vi "Circus Config Param - Core.vi"(6 "Load":bool, 8 "error in (no error)":errorcluster, 11 "Parameter Name":string) -> (0 "error out":errorcluster, 3 "Output":string)   [LabVIEW 2026, in "TALOS.lvlib"]
doc: "This VI stores in memory all the AEgIS configuration parameters loaded at startup from AEgIS_Config_Param.ini. It only runs when the VI is called from the PPL version of TALOS."
uses:
  TALOS.lvlib
  Ancestor/Ancestor/Ancestor.lvclass/Ancestor.ctl
  FGV/Error Memory/Get Error Description.vi
  Get PC name.vi
  Ancestor/Ancestor/Read ID.vi
  Get Class Name.vi
  <vilib>/Utility/error.llb/Clear Errors.vi
  FGV/Error Memory/Error Memory Core.vi
  <vilib>/AdvancedString/Delimited String to 1D String Array.vi
  <vilib>/AdvancedString/Delimited String to 1D String Array (string).vi
  FGV/Error Memory/Error Crt Lvl checker.vi
  FGV/Error Memory/Error Memory Core.vi/40c8088d-b597-4017-91af-faa98e00292e.vi
  FGV/Error Memory/Error Memory Core.vi/d4a3ab98-063c-4e44-b43d-fbdcfe6c2be2.vi
  Global Memory.vi
  <vilib>/Utility/LVClass/Get LV Class Name.vi
  TALOS Root path.vi
  Read CSV worksheet.vi
  Global Constants.vi
  <vilib>/Utility/error.llb/General Error Handler.vi
  <vilib>/Utility/config.llb/Read Key (String).vi
  Ancestor/Ancestor/Ancestor.lvclass
  <vilib>/Comparison/Equal/Equal Functor/Equal Functor.lvclass
  <vilib>/Utility/config.llb/NI_LVConfig.lvlib
panel:
  out "key names":string[][](array[string])
  out "section names":string[](array[string])
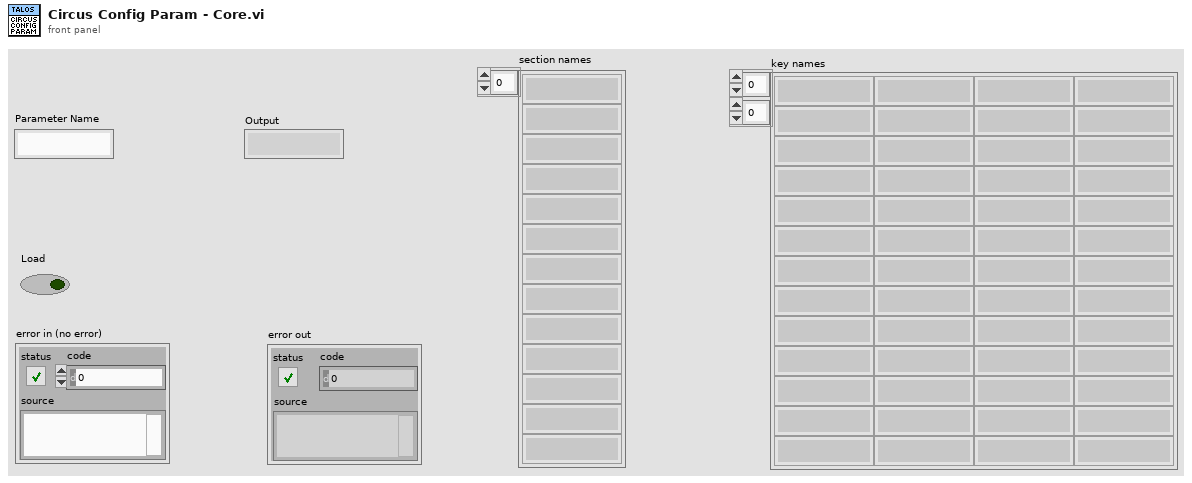
[diagram p1: front panel]
types:
  T1 = typedef "NI_LVConfig.lvlib/Config Data RefNum.ctl" = refnum<k1>
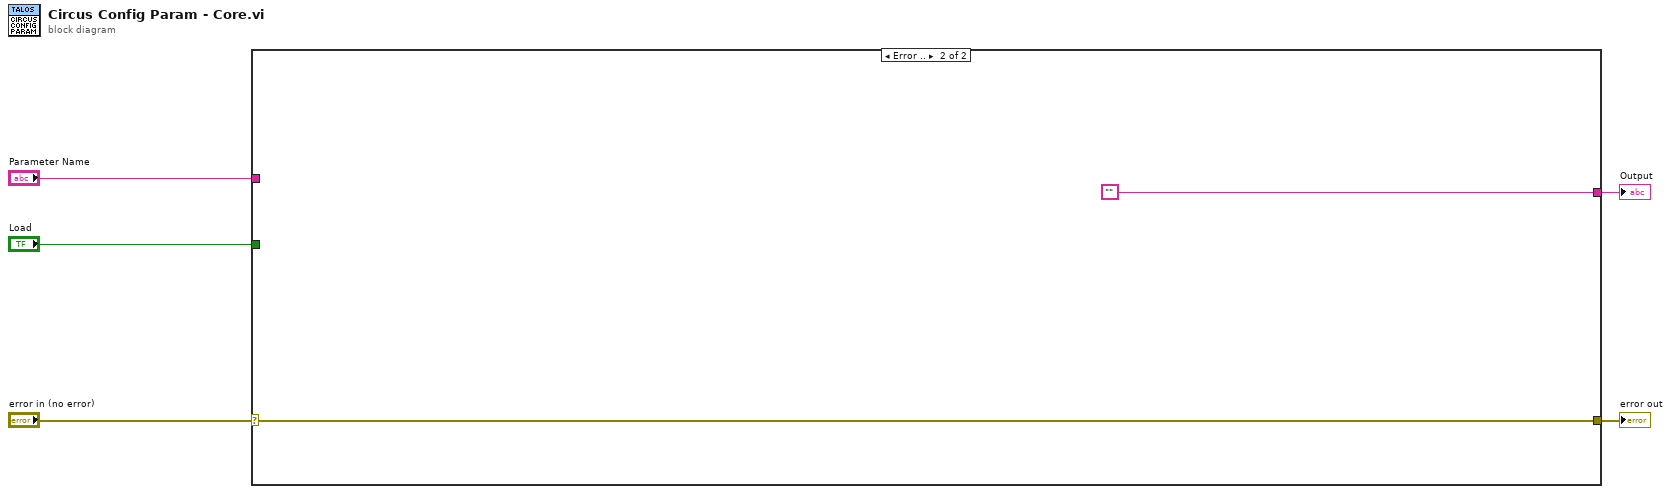
[diagram p0: block diagram]
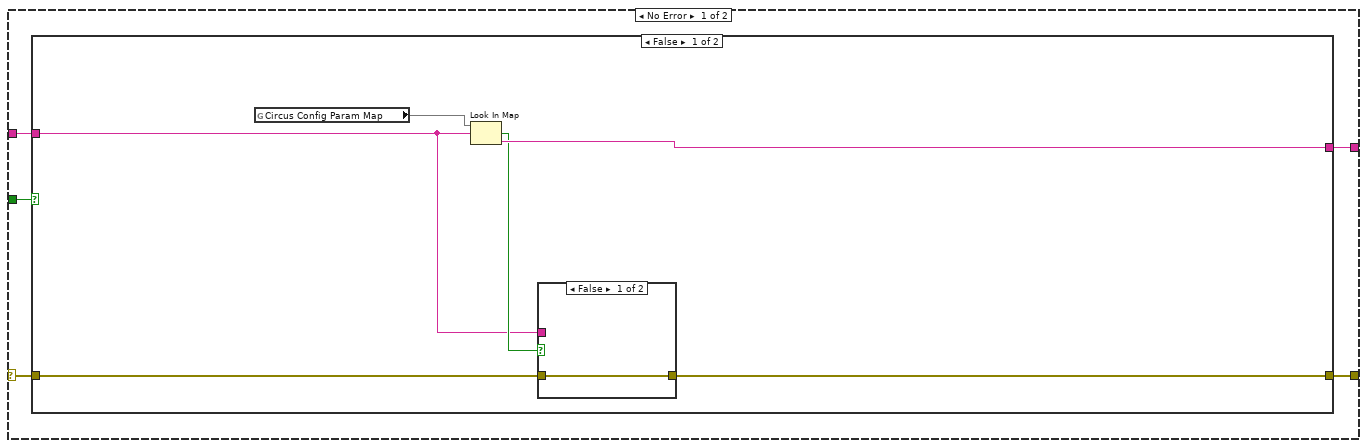
[diagram p2: hidden frame]
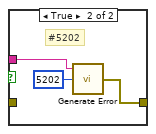
[diagram p3: hidden frame]
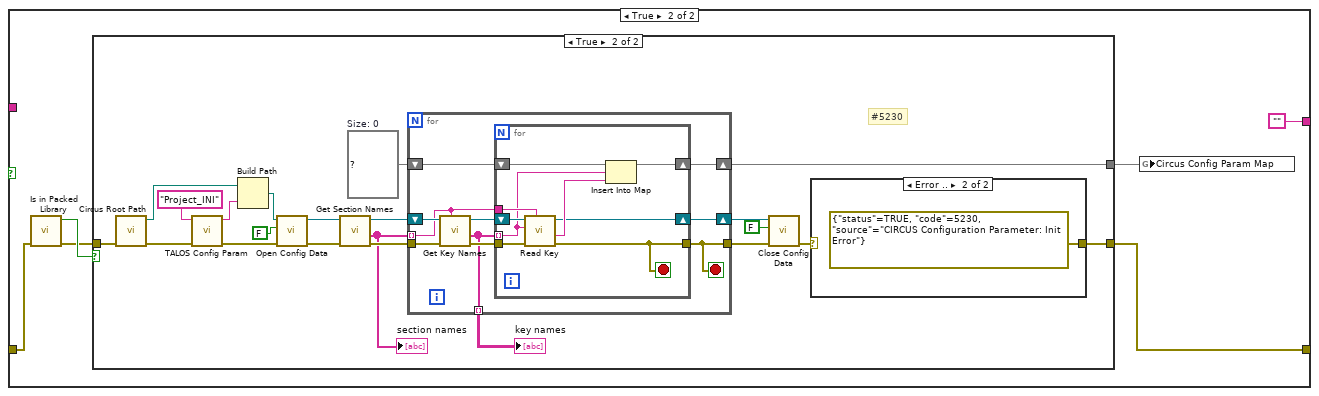
[diagram p4: hidden frame]
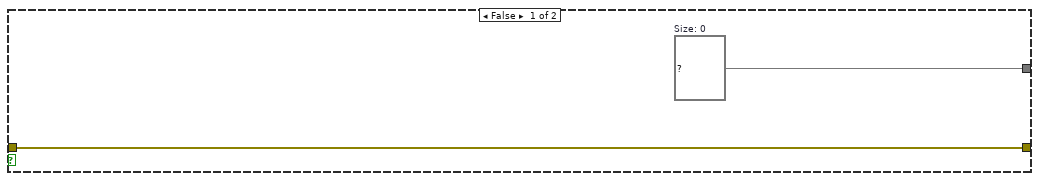
[diagram p5: hidden frame]
diagram:
  n1 = case shown="Error .." "error in (no error)" {
    selector: "error in (no error)" -> [w6 w72]
    tunnel: "Load" -> [w10 _]
    tunnel: [w9 w72] -> w4
    tunnel: [w8 "" ("Empty String Constant")] -> w3
    tunnel: "Parameter Name" -> [w7 _]
    frame No Error {
      n2 = case shown="False" w10 {
        tunnel: w6 -> [w14 w21]
        tunnel: [w13 w26] -> w9
        tunnel: [w16 "" ("Output")] -> w8
        tunnel: w7 -> [w11 _]
        frame False {
          n3 = global read "Global Memory.vi" "Circus Config Param Map"() -> (w12:map{string, string})
          n4 = Look In Map(map=w12, key=w11) -> (key not found?=w15:bool, value=w16:string)  [unwired: 1 in]
          n5 = case shown="False" w15 {
            tunnel: [w17 w19] -> w13
            tunnel: w14 -> [w17 _]
            tunnel: w11 -> [_ w18]
            frame False {
            }
            frame True {
              # "#5202"
              n6 = call "Generate Error.vi"("Optional String"=w18, "Error Code"=5202) -> ("error out"=w19:errorcluster)  [unwired: 5 in]
            }
          }
        }
        frame True {
          n7 = call "Is in Packed Library.vi"("error in (no error)"=w21) -> ("error out"=w22:errorcluster, "Is In Packed Library"=w23:bool)  [unwired: 9 in]
          n8 = case shown="True" w23 {
            tunnel: [w28 w33] -> w26
            tunnel: w22 -> [w28 w36]
            tunnel: [w27 w35] -> w24
            frame False {
              w27 = map{string, string} {}  # Size: 0
            }
            frame True {
              w37 = map{string, string} {}  # Size: 0
              # "#5230"
              n9 = call "Circus Root Path.vi"("error in (no error)"=w36) -> ("error out"=w31:errorcluster, "Circus Root Path"=w38:path)  [unwired: 9 in]
              n10 = call "TALOS Config Param.vi"("error in (no error)"=w31, "Parameter Name"="Project_INI") -> ("error out"=w29:errorcluster, "Output"=w30:string)  [unwired: 8 in]
              n11 = Build Path(base path=w38, name or relative path=w30) -> (appended path=w39:path)
              n12 = call <vilib>:"Open Config Data.vi"("error in (no error)"=w29, "create file if necessary (T)"=FALSE, "configuration file path"=w39) -> ("error out"=w48:errorcluster, "refnum"=w47:T1)  [unwired: 6 in, 1 out]
              n13 = call <vilib>:"Get Section Names.vi"("error in (no error)"=w48, "refnum"=w47) -> ("error out"=w45:errorcluster, "section names"=w44:string[], "refnum out"=w46:T1)  [unwired: 7 in]
              "section names" <- w44
              n14 = for {
                tunnel: w45 -> [w60]
                tunnel: w44 -> [w57] mode=indexing
                tunnel: [w56] -> w43 mode=indexing
                tunnel: [w52] -> w42
                shift-right: [w55] -> w35
                shift-left: w37 -> [w54]
                shift-right: [w53] -> w41
                shift-left: w46 -> [w61]
                stop <- w52 stop-if-true
                n15 = call <vilib>:"Get Key Names.vi"("section"=w57, "error in (no error)"=w60, "refnum"=w61) -> ("error out"=w58:errorcluster, "key names"=w56:string[], "refnum out"=w59:T1)  [unwired: 5 in, 1 out]
                n16 = for {
                  tunnel: w58 -> [w69]
                  tunnel: w57 -> [w68]
                  tunnel: w56 -> [w67] mode=indexing
                  tunnel: [w62] -> w52
                  shift-right: [w65] -> w55
                  shift-left: w54 -> [w64]
                  shift-right: [w63] -> w53
                  shift-left: w59 -> [w70]
                  stop <- w62 stop-if-true
                  n17 = call-poly <vilib>:"Read Key.vi"("section"=w68, "error in (no error)"=w69, "key"=w67, "refnum"=w70) -> ("error out"=w62:errorcluster, "value"=w66:string, "refnum out"=w63:T1)  [unwired: 4 in, 1 out]
                  n18 = Insert Into Map(map in=w64, key=w67, value=w66) -> (map out=w65:map{string, string})  [unwired: 2 out]
                }
              }
              "key names" <- w43
              n19 = call <vilib>:"Close Config Data.vi"("error in (no error)"=w42, "write file if changed (T)"=FALSE, "refnum"=w41) -> ("error out"=w34:errorcluster)  [unwired: 7 in, 1 out]
              n20 = case shown="Error .." w34 {
                selector: w34 -> [w50 _]
                tunnel: [w50 errorcluster {"status"=TRUE, "code"=5230, "source"="CIRCUS Configuration Parameter: Init Error"} ("error IO")] -> w33
                frame No Error {
                }
                frame Error {
                }
              }
            }
          }
          n21 = global write "Global Memory.vi" "Circus Config Param Map"(w24) -> ()
        }
      }
    }
    frame Error {
    }
  }
  "error out" <- w4
  "Output" <- w3
